vi "QColor.vi"(4 "a (255)":i32=255, 6 "b":i32, 8 "Error In":errorcluster, 9 "g":i32, 10 "r":i32) -> (0 "Error Out":errorcluster, 3 "New QColor":refnum<class "QColor.lvclass">)   [LabVIEW 2014, in "QColor.lvclass"]
doc: "LabVIEW-specific documentation is not yet available. See <b>http://doc.qt.io/qt-5/QColor.html#QColor</b>"
uses:
  QColor.lvclass
  LQ Core/LQSerialData/LQSerialData.lvclass/LQSerialData.ctl
  LQ Core/LQ Core.lvlib
  LQ Core/LQSerialData/LQSerialData.lvclass
panel:
  # "Copyright (c) 2016 Sze Howe Koh\n\nThis Source Code Form is subject to the terms of the Mozilla Public\nLicense, v. 2.0. If a copy of the MPL was not distributed with this\nfile, You can obtain one at http://mozilla.org/MPL/2.0/."
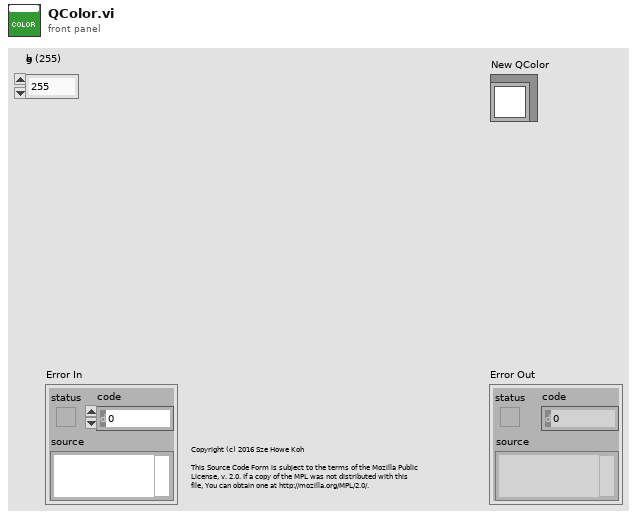
[diagram p1: front panel]
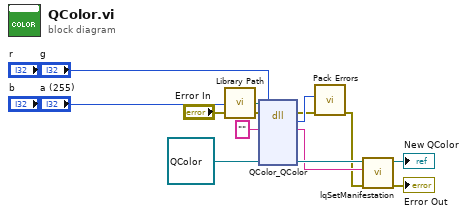
[diagram p0: block diagram]
diagram:
  n1 = call "Library Path.vi"() -> ("Library Path"=w9:path)
  n2 = dll-call lib="?" fn="QColor_QColor"(path in=w9, error in="Error In", "_retVal"="", "r"="r", "g"="g", "b"="b", "a"="a (255)") -> (error out=w7:errorcluster, w8:i32, "_retVal"=w10:string)  [unwired: 5 in, 1 out]
  n3 = call "Pack Errors.vi"("Error In"=w7, "Error Code"=w8) -> ("Error Out"=w6:errorcluster)  [unwired: 9 in]
  n4 = call "lqSetManifestation.vi"("Error In"=w6, "Manifestation"=w10, "LQSerialData in"=refnum<class "QColor.lvclass"> refnum ("QColor")) -> ("Error Out"=→"Error Out":errorcluster, "LQSerialData out"=→"New QColor":refnum<class "QColor.lvclass">)  [unwired: 7 in]
